vi "Handle getAll.vi"(8 "error in (no error)":errorcluster, 11 "Example Instrument in":refnum<class "Instrument.Element2.lvclass">) -> (0 "error out":errorcluster, 2 "getAll":variant, 3 "Example Instrument out":refnum<class "Instrument.Element2.lvclass">)   [LabVIEW 2019, in "Instrument.Element2.lvclass"]
uses:
  Instrument.Element2.lvclass
  Typedefs/Instrument.Element2.getAll--Cluster.ctl
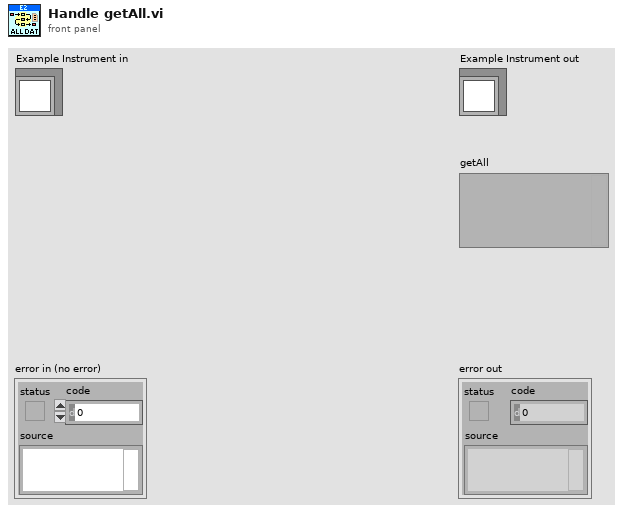
[diagram p1: front panel]
types:
  T1 = typedef "Instrument.Element2.lvclass/Instrument.Element2.getAll--Cluster.ctl" = cluster{"Power":dbl, "Laser Status":string, "Pump Status":string}
  T2 = cluster{"Firmware":string, "[1]":string, "Serial No.":string, "[3]":string, "Laser Hrs.":string, "Year (YYYY)":string, "Month (MM)":string, "Date (DD)":string, "Hours (hh)":string, "Minutes (mm)":string, "Seconds (ss)":string, "[11]":string, "[12]":string, "Laser Status":string, "[14]":string, "Pump Status":string, "[16]":string, "[17]":string, "[18]":string, "[19]":string, "[20]":string, "[21]":string, "[22]":string, "[23]":string, "[24]":string, "[25]":string, "[26]":string, "Pico Speed":string, "Pico #":string, "[29]":string, "[30]":string, "[31]":string, "[32]":string, "[33]":string, "[34]":string, "[35]":string, "[36]":string, "[37]":string, "[38]":string, "[39]":string, "[40]":string, "[41]":string, "[42]":string, "[43]":string, "[44]":string, "[45]":string, "[46]":string, "[47]":string, "[48]":string, "[49]":string, "[50]":string, "[51]":string, "[52]":string, "[53]":string, "[54]":string, "[55]":string, "[56]":string, "[57]":string, "[58]":string, "[59]":string, "[60]":string, "[61]":string, "[62]":string, "[63]":string, "[64]":string, "[65]":string, "[66]":string, "[67]":string, "[68]":string, "[69]":string, "[70]":string, "[71]":string, "[72]":string, "[73]":string, "[74]":string, "Pump Laser 1":string, "Pump Laser 2":string, "Pump Laser 3":string, "Pump Laser 4":string, "Pump Laser 5":string, "[80]":string, "[81]":string, "[82]":string, "[83]":string, "[84]":string, "Diode Current Set":string, "Diode Current Actual":string, "[87]":string, "Power":string, "[89]":string, "[90]":string, "[91]":string, "Temp: Pump Chassis":string, "Temp: Pump Diodes":string, "Temp: Pump Tower":string, "Temp: Pump PCB":string, "SHG Point":string, "[97]":string, "[98]":string, "[99]":string, "[100]":string, "[101]":string, "[102]":string, "Spectrometer: Int. time":string, "[104]":string, "[105]":string, "[106]":string, "Starter: Duration":string, "Starter: Voltage":string, "Starter: PWM Mode":string, "Starter: Duty Cycle":string, "PowSensCtrlLoop: Kp":string, "PowSensCtrlLoop: Ki":string, "Cycle Time":string, "Max Pump Current":string, "Loop Status":string, "CrysPos: Move Interval":string, "CrysPos: Pico Steps":string, "CrysPos: Step Direction":string, "CrysPos: Max Moves":string, "CrysPos: Last Move":string, "CrysPos: Moves Done":string, "Temp: Control Unit":string, "Temp: Laser Head Pos 1":string, "Temp: Laser Head Pos 2":string, "[125]":string, "[126]":string, "[127]":string, "[128]":string, "[129]":string, "[130]":string, "[131]":string, "[132]":string, "[133]":string, "[134]":string, "[135]":string, "[136]":string, "[137]":string, "[138]":string, "[139]":string, "[140]":string, "[141]":string, "Wedge Control Counter":string, "[143]":string}
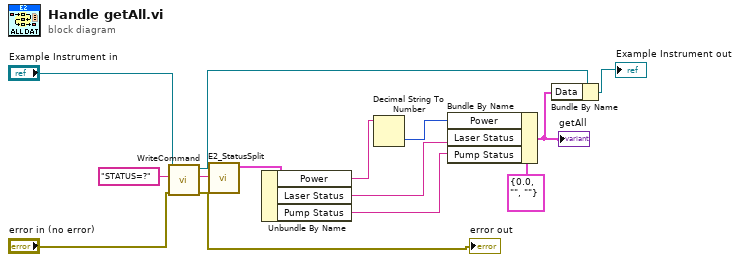
[diagram p0: block diagram]
diagram:
  n1 = call "WriteCommand.vi"("error in (no error)"="error in (no error)", "Command"="STATUS=?" ("Write Buffer"), "Instrument.Element2 in"="Example Instrument in") -> ("error out"=→"error out":errorcluster, "Read Buffer"=w12:string, "Instrument.Element2 out"=w5:refnum<class "Instrument.Element2.lvclass">)  [unwired: 6 in]
  n2 = call "E2_StatusSplit.vi"("Input String"=w12) -> ("Output Cluster"=w11:T2)  [unwired: 10 in]
  n3 = Unbundle By Name(w11) -> ("Power"=w9:string, "Laser Status"=w7:string, "Pump Status"=w6:string)
  n4 = Decimal String To Number(string=w9) -> (number=w8:i32)  [unwired: 2 in, 1 out]
  n5 = Bundle By Name(cluster=T1 {"Power"=0.0, "Laser Status"="", "Pump Status"=""} ("getAll"), "Power"=w8, "Laser Status"=w7, "Pump Status"=w6) -> (w3:T1)
  "getAll" <- w3
  n6 = Bundle By Name(cluster=w5, "Data"=w3) -> (→"Example Instrument out":refnum<class "Instrument.Element2.lvclass">)
